vi "Main_control_sistem.vi"(9 "Numeric":i32, 10 "Measurement in":dbl, 11 "read buffer":string) -> (2 "Measurement out":dbl, 3 "Action":string)   [LabVIEW 2015]
uses:
  Read_from_serial_and_create/Test_Code/Global 5.vi
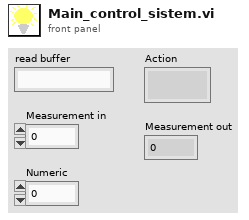
[diagram p1: front panel]
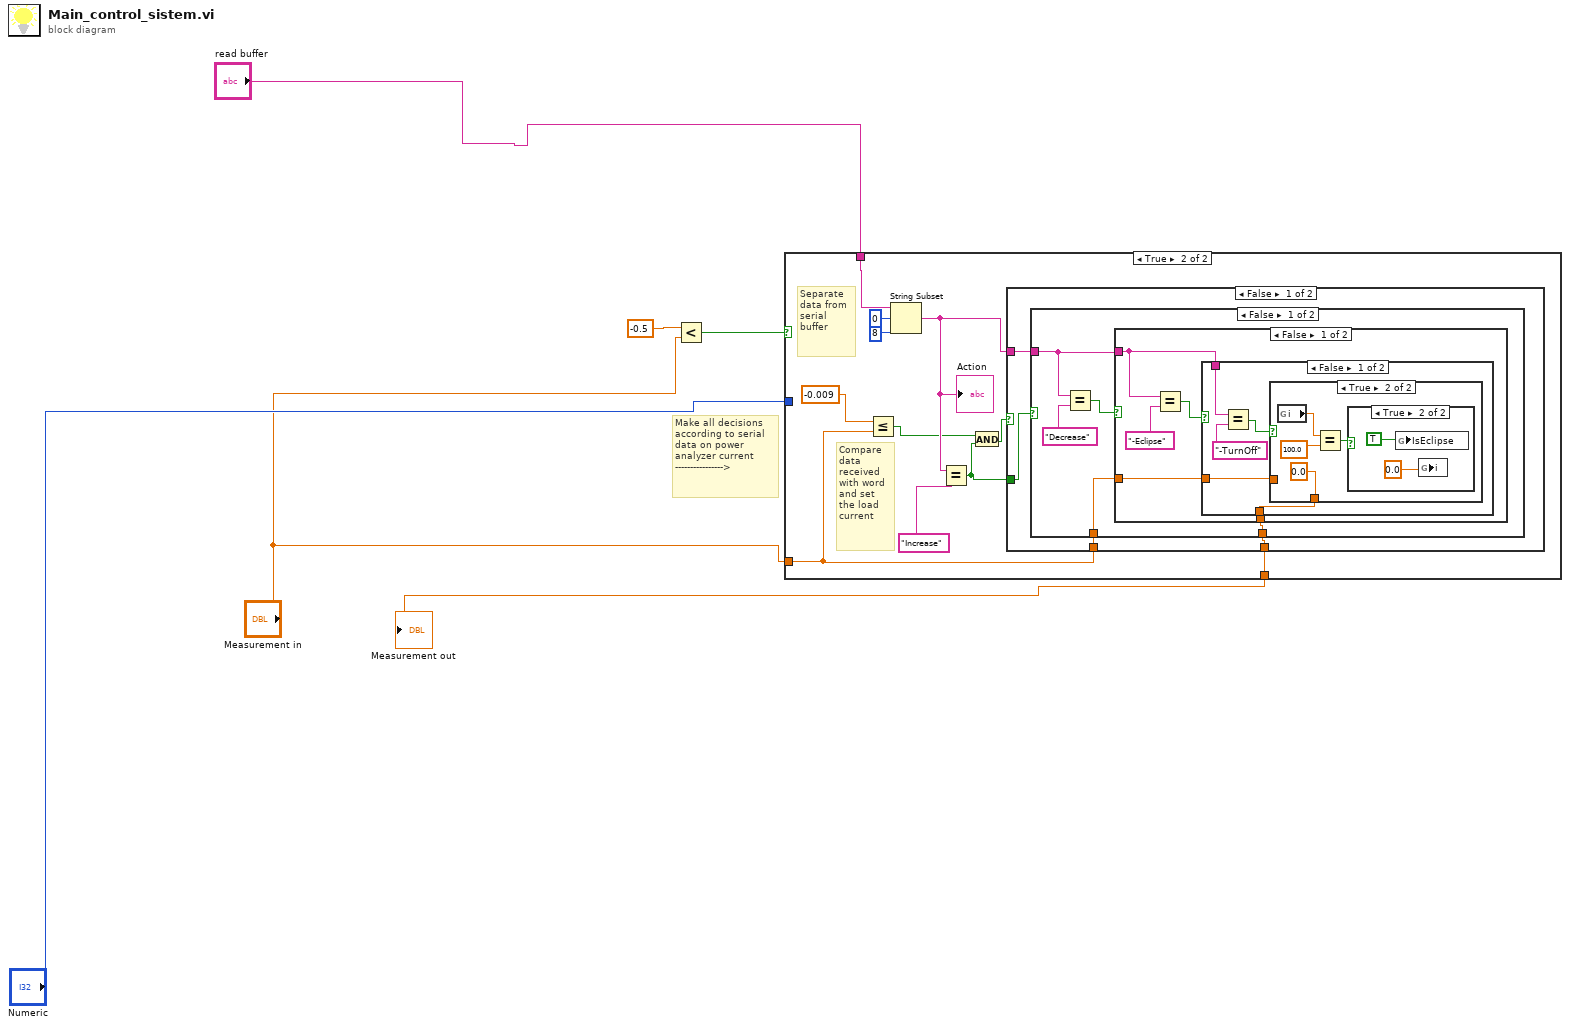
[diagram p0: block diagram]
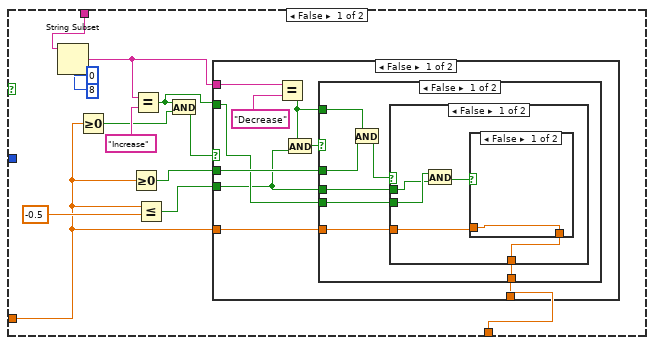
[diagram p2: hidden frame]
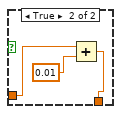
[diagram p3: hidden frame]
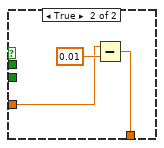
[diagram p4: hidden frame]
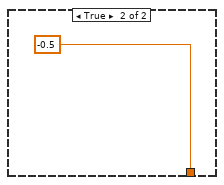
[diagram p5: hidden frame]
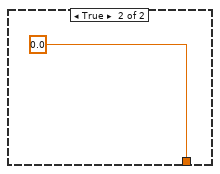
[diagram p6: hidden frame]
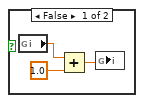
[diagram p8: hidden frame]
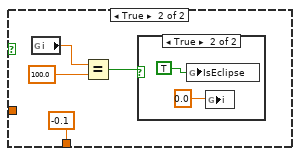
[diagram p9: hidden frame]
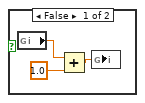
[diagram p10: hidden frame]
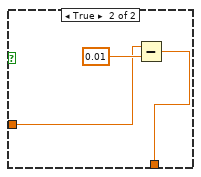
[diagram p11: hidden frame]
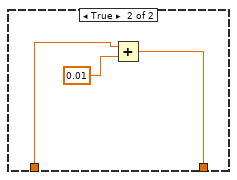
[diagram p12: hidden frame]
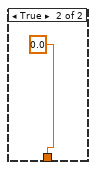
[diagram p13: hidden frame]
diagram:
  # "Make all decisions according to serial data on power analyzer current\n---------------->"
  n1 = Less?(x=-0.5, y="Measurement in") -> (x < y?=w2:bool)
  n2 = case shown="True" w2 {
    tunnel: [w19 w60] -> w6
    tunnel: "Measurement in" -> [w8 w53]
    tunnel: "read buffer" -> [w12 w58]
    tunnel: "Numeric" -> [_ _]
    frame False {
      n3 = String Subset(string=w12, offset (0)=0, length (rest)=8 ("length (rest)")) -> (substring=w11:string)
      n4 = Greater Or Equal To 0?(x=w8) -> (x >= 0?=w7:bool)
      n5 = Greater Or Equal To 0?(x=w8) -> (x >= 0?=w10:bool)
      n6 = Equal?(x=w11, y="Increase") -> (x = y?=w9:bool)
      n7 = Less Or Equal?(x=w8, y=-0.5) -> (x <= y?=w16:bool)
      n8 = And(x=w9, y=w7) -> (x .and. y?=w18:bool)
      n9 = case shown="False" w18 {
        tunnel: [w25 0.0] -> w19
        tunnel: w16 -> [w20 _]
        tunnel: w11 -> [w27 _]
        tunnel: w10 -> [w23 _]
        tunnel: w8 -> [w22 _]
        tunnel: w9 -> [w21 _]
        frame False {
          n10 = Equal?(x=w27, y="Decrease") -> (x = y?=w24:bool)
          n11 = And(x=w24, y=w20) -> (x .and. y?=w28:bool)
          n12 = case shown="False" w28 {
            tunnel: [w32 -0.5] -> w25
            tunnel: w24 -> [w34 _]
            tunnel: w23 -> [w33 _]
            tunnel: w22 -> [w31 _]
            tunnel: w21 -> [w30 _]
            tunnel: w20 -> [w29 _]
            frame False {
              n13 = And(x=w34, y=w33) -> (x .and. y?=w35:bool)
              n14 = case shown="False" w35 {
                tunnel: [w37 w47] -> w32
                tunnel: w31 -> [w36 w45]
                tunnel: w30 -> [w40 _]
                tunnel: w29 -> [w39 _]
                frame False {
                  n15 = And(x=w40, y=w39) -> (x .and. y?=w38:bool)
                  n16 = case shown="False" w38 {
                    tunnel: [w41 w44] -> w37
                    tunnel: w36 -> [w41 w43]
                    frame False {
                    }
                    frame True {
                      n17 = Add(x=w43, y=0.01) -> (x+y=w44:dbl)
                    }
                  }
                }
                frame True {
                  n18 = Subtract(x=w45, y=0.01) -> (x-y=w47:dbl)
                }
              }
            }
            frame True {
            }
          }
        }
        frame True {
        }
      }
    }
    frame True {
      # "Compare data received with word and set the load current"
      # "Separate data from serial buffer"
      n19 = Less Or Equal?(x=-0.009, y=w53) -> (x <= y?=w50:bool)
      n20 = String Subset(string=w58, offset (0)=0, length (rest)=8 ("length (rest)")) -> (substring=w55:string)
      "Action" <- w55
      n21 = Equal?(x=w55, y="Increase") -> (x = y?=w52:bool)
      n22 = And(x=w50, y=w52) -> (x .and. y?=w51:bool)
      n23 = case shown="False" w51 {
        tunnel: [w64 0.0 ("Measurement")] -> w60
        tunnel: w52 -> [w63 _]
        tunnel: w53 -> [w62 _]
        tunnel: w55 -> [w61 _]
        frame False {
          n24 = case shown="False" w63 {
            tunnel: [w69 w103] -> w64
            tunnel: w61 -> [w65 _]
            tunnel: w62 -> [w66 w102]
            frame False {
              n25 = Equal?(x=w65, y="Decrease") -> (x = y?=w68:bool)
              n26 = case shown="False" w68 {
                tunnel: [w72 w100] -> w69
                tunnel: w66 -> [w71 w99]
                tunnel: w65 -> [w70 _]
                frame False {
                  n27 = Equal?(x=w70, y="-Eclipse") -> (x = y?=w74:bool)
                  n28 = case shown="False" w74 {
                    tunnel: [w76 -0.1] -> w72
                    tunnel: w71 -> [w75 _]
                    tunnel: w70 -> [w78 _]
                    frame False {
                      n29 = Equal?(x=w78, y="-TurnOff") -> (x = y?=w79:bool)
                      n30 = case shown="True" w79 {
                        tunnel: [w80 0.0 ("x")] -> w76
                        tunnel: w75 -> [w80 _]
                        frame False {
                        }
                        frame True {
                          n31 = global read "Global 5.vi" "i"() -> (w81:dbl)
                          n32 = Equal?(x=w81, y=100.0) -> (x = y?=w83:bool)
                          n33 = case shown="True" w83 {
                            frame False {
                              n34 = global read "Global 5.vi" "i"() -> (w85:dbl)
                              n35 = Add(x=w85, y=1.0) -> (x+y=w86:dbl)
                              n36 = global write "Global 5.vi" "i"(w86) -> ()
                            }
                            frame True {
                              n37 = global write "Global 5.vi" "IsEclipse"(TRUE ("Boolean")) -> ()
                              n38 = global write "Global 5.vi" "i"(0.0 ("i")) -> ()
                            }
                          }
                        }
                      }
                    }
                    frame True {
                      n39 = global read "Global 5.vi" "i"() -> (w90:dbl)
                      n40 = Equal?(x=w90, y=100.0) -> (x = y?=w92:bool)
                      n41 = case shown="True" w92 {
                        frame False {
                          n42 = global read "Global 5.vi" "i"() -> (w95:dbl)
                          n43 = Add(x=w95, y=1.0) -> (x+y=w94:dbl)
                          n44 = global write "Global 5.vi" "i"(w94) -> ()
                        }
                        frame True {
                          n45 = global write "Global 5.vi" "IsEclipse"(TRUE ("Boolean")) -> ()
                          n46 = global write "Global 5.vi" "i"(0.0 ("i")) -> ()
                        }
                      }
                    }
                  }
                }
                frame True {
                  n47 = Subtract(x=w99, y=0.01) -> (x-y=w100:dbl)
                }
              }
            }
            frame True {
              n48 = Add(x=w102, y=0.01) -> (x+y=w103:dbl)
            }
          }
        }
        frame True {
        }
      }
    }
  }
  "Measurement out" <- w6
